vi "Sync In (TDM).vi"(5 "start delay (0)":u8, 6 "channel count (2)":u8=2, 7 "data sample edge (rising)":enum16{"rising", "falling"}(ring), 8 "receive":bool, 9 "prev transfer done":bool, 10 "frame sync in":bool, 11 "clock in":bool) -> (0 "latch config":bool, 1 "force output":bool, 2 "start read":bool)   [LabVIEW 2013, in "I2S-TDM.lvlib"]
uses:
  I2S-TDM.lvlib
  Controls/frame sync states.ctl
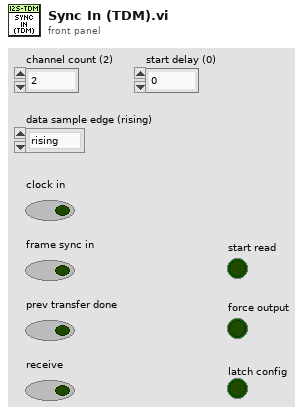
[diagram p1: front panel]
types:
  T1 = typedef "I2S-TDM.lvlib/frame sync states.ctl" = enum16{"idle", "pre-transfer", "transfer"}
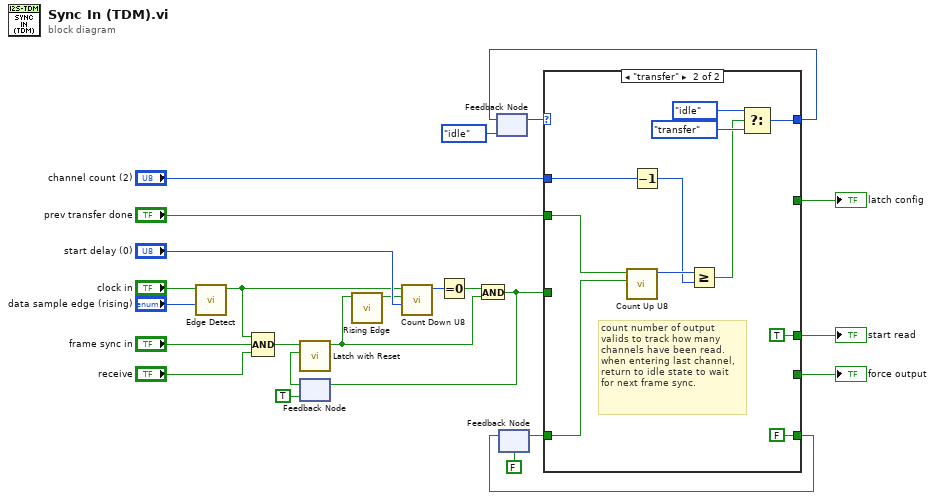
[diagram p0: block diagram]
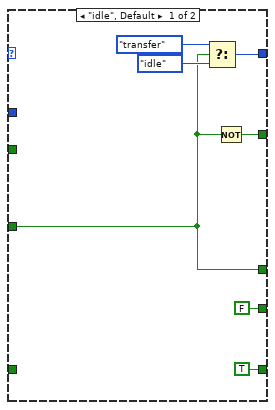
[diagram p2: hidden frame]
diagram:
  n1 = call "Edge Detect.vi"("edge (rising)"="data sample edge (rising)", "signal in"="clock in") -> ("edge detected?"=w2:bool)  [unwired: 9 in]
  n2 = Compound Arithmetic op=AND(w2, "frame sync in", "receive") -> (w4:bool)
  n3 = feedback #1(TRUE) -> (w11:bool)
  n4 = call "Latch with Reset.vi"("reset"=w11, "signal"=w4) -> ("latched signal"=w1:bool)  [unwired: 9 in]
  n5 = call "Rising Edge.vi"("signal in"=w1) -> ("rising edge?"=w3:bool)  [unwired: 10 in]
  n6 = call "Count Down U8.vi"("reset value"="start delay (0)", "reset"=w3, "decrement"=w2) -> ("count"=w12:u8)  [unwired: 8 in]
  n7 = Equal To 0?(x=w12) -> (x = 0?=w9:bool)
  n8 = And(x=w9, y=w1) -> (x .and. y?=w6:bool)
  n9 = feedback-in #1(w6) -> ()
  n10 = feedback #2(frame_sync_states."idle") -> (w24:T1)
  n11 = feedback #3(FALSE) -> (w16:bool)
  n12 = case shown="\"transfer\"" w24 {
    tunnel: [w30 w35] -> w13
    tunnel: [w26 TRUE ("edge detected?")] -> w21
    tunnel: "channel count (2)" -> [_ w42]
    tunnel: [w27 _] -> w22
    tunnel: [FALSE ("latched signal") _] -> w20
    tunnel: [TRUE FALSE] -> w15
    tunnel: w16 -> [_ w41]
    tunnel: "prev transfer done" -> [_ w40]
    tunnel: w6 -> [w26 _]
    frame "idle", Default {
      n13 = Select(t=frame_sync_states."transfer", s=w26, f=frame_sync_states."idle") -> (s? t:f=w30:T1)
      n14 = Not(x=w26) -> (.not. x?=w27:bool)
    }
    frame "transfer" {
      # "count number of output valids to track how many channels have been read. when entering last channel, return to idle state to wait for next frame sync."
      n15 = call "Count Up U8.vi"("reset (F)"=w41, "increment"=w40) -> ("count"=w38:u8)  [unwired: 9 in]
      n16 = Decrement(x=w42) -> (x-1=w33:u8)
      n17 = Greater Or Equal?(x=w38, y=w33) -> (x >= y?=w34:bool)
      n18 = Select(t=frame_sync_states."idle", s=w34, f=frame_sync_states."transfer") -> (s? t:f=w35:T1)
    }
  }
  "start read" <- w21
  "latch config" <- w22
  "force output" <- w20
  n19 = feedback-in #2(w13) -> ()
  n20 = feedback-in #3(w15) -> ()
